vi "CycleVoltammetry.vi"() -> ()   [LabVIEW 2014]
uses:
  <vilib>/Instr/_visa.llb/VISA Configure Serial Port (Instr).vi
panel:
  in  "Combo Box":string(combo)
  out "R":dbl
  in  "stop":bool
  in  "file path (use dialog)":path
  in  "Title of experiment":string
  out "当前电流（A）":dbl
  out "Error buffer":string
  in  "Quiet Time Before SCAN(s)":dbl
  in  "VISA resource name":refnum<visa-resource-name>
  out "millisecond timer value 2":u32
  out "Index":dbl
  out "当前电压（V）":dbl
  in  "正向/反向(点亮)":bool
  out "V":dbl(graph)
  out "I":dbl(graph)
  out "I-U Graph":cluster{dbl[], dbl[]}(graph)
  in  "悬停（Pause）":bool
  out "Boolean":bool
  out "Run time":u32
  out "Program statement":string
  in  "Quiet Time(s)":dbl
  in  "反向/正向扫描(反向点亮)":bool caption="反向扫描"
  in  "Initial Voltage (起始电压\\V)":dbl
  in  "Sweep Segments(循环次数\\Times)":dbl
  out "Qutie Time （延时时间\\ms)":dbl
  in  "Low Voltage(最小电压\\V)":dbl
  in  "High Voltage(最大电压\\V)":dbl
  in  "Scan Rate(进步电压 V/Step）":dbl
  in  "Final Voltage(终止电压\\V)":dbl
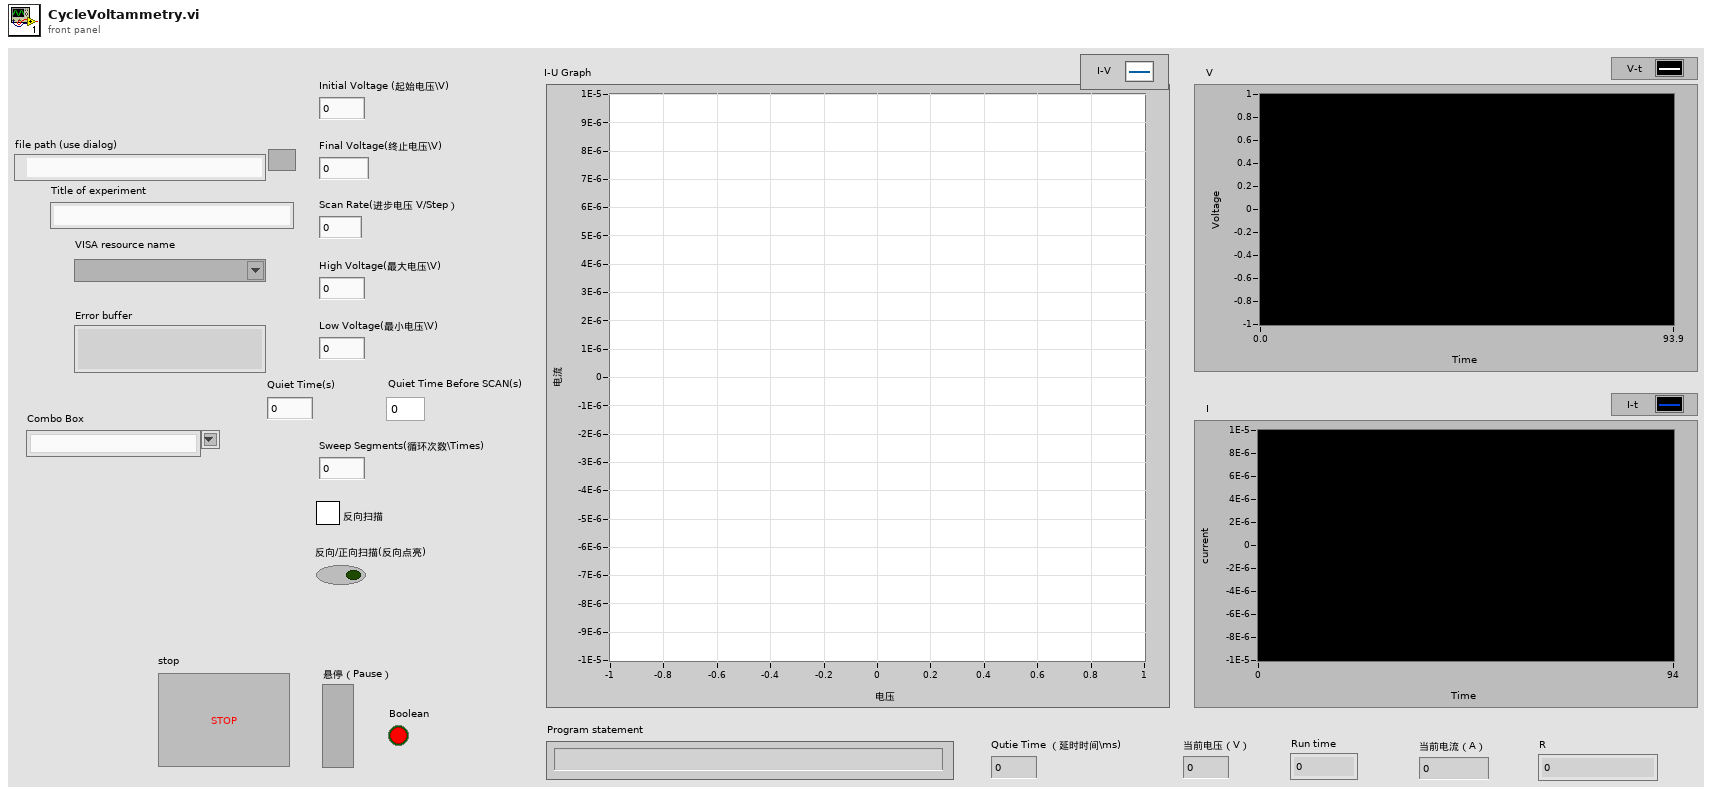
[diagram p1: front panel]
types:
  T1 = enum16{"open", "replace", "create", "open or create", "replace or create", "replace or create with confirmation"}
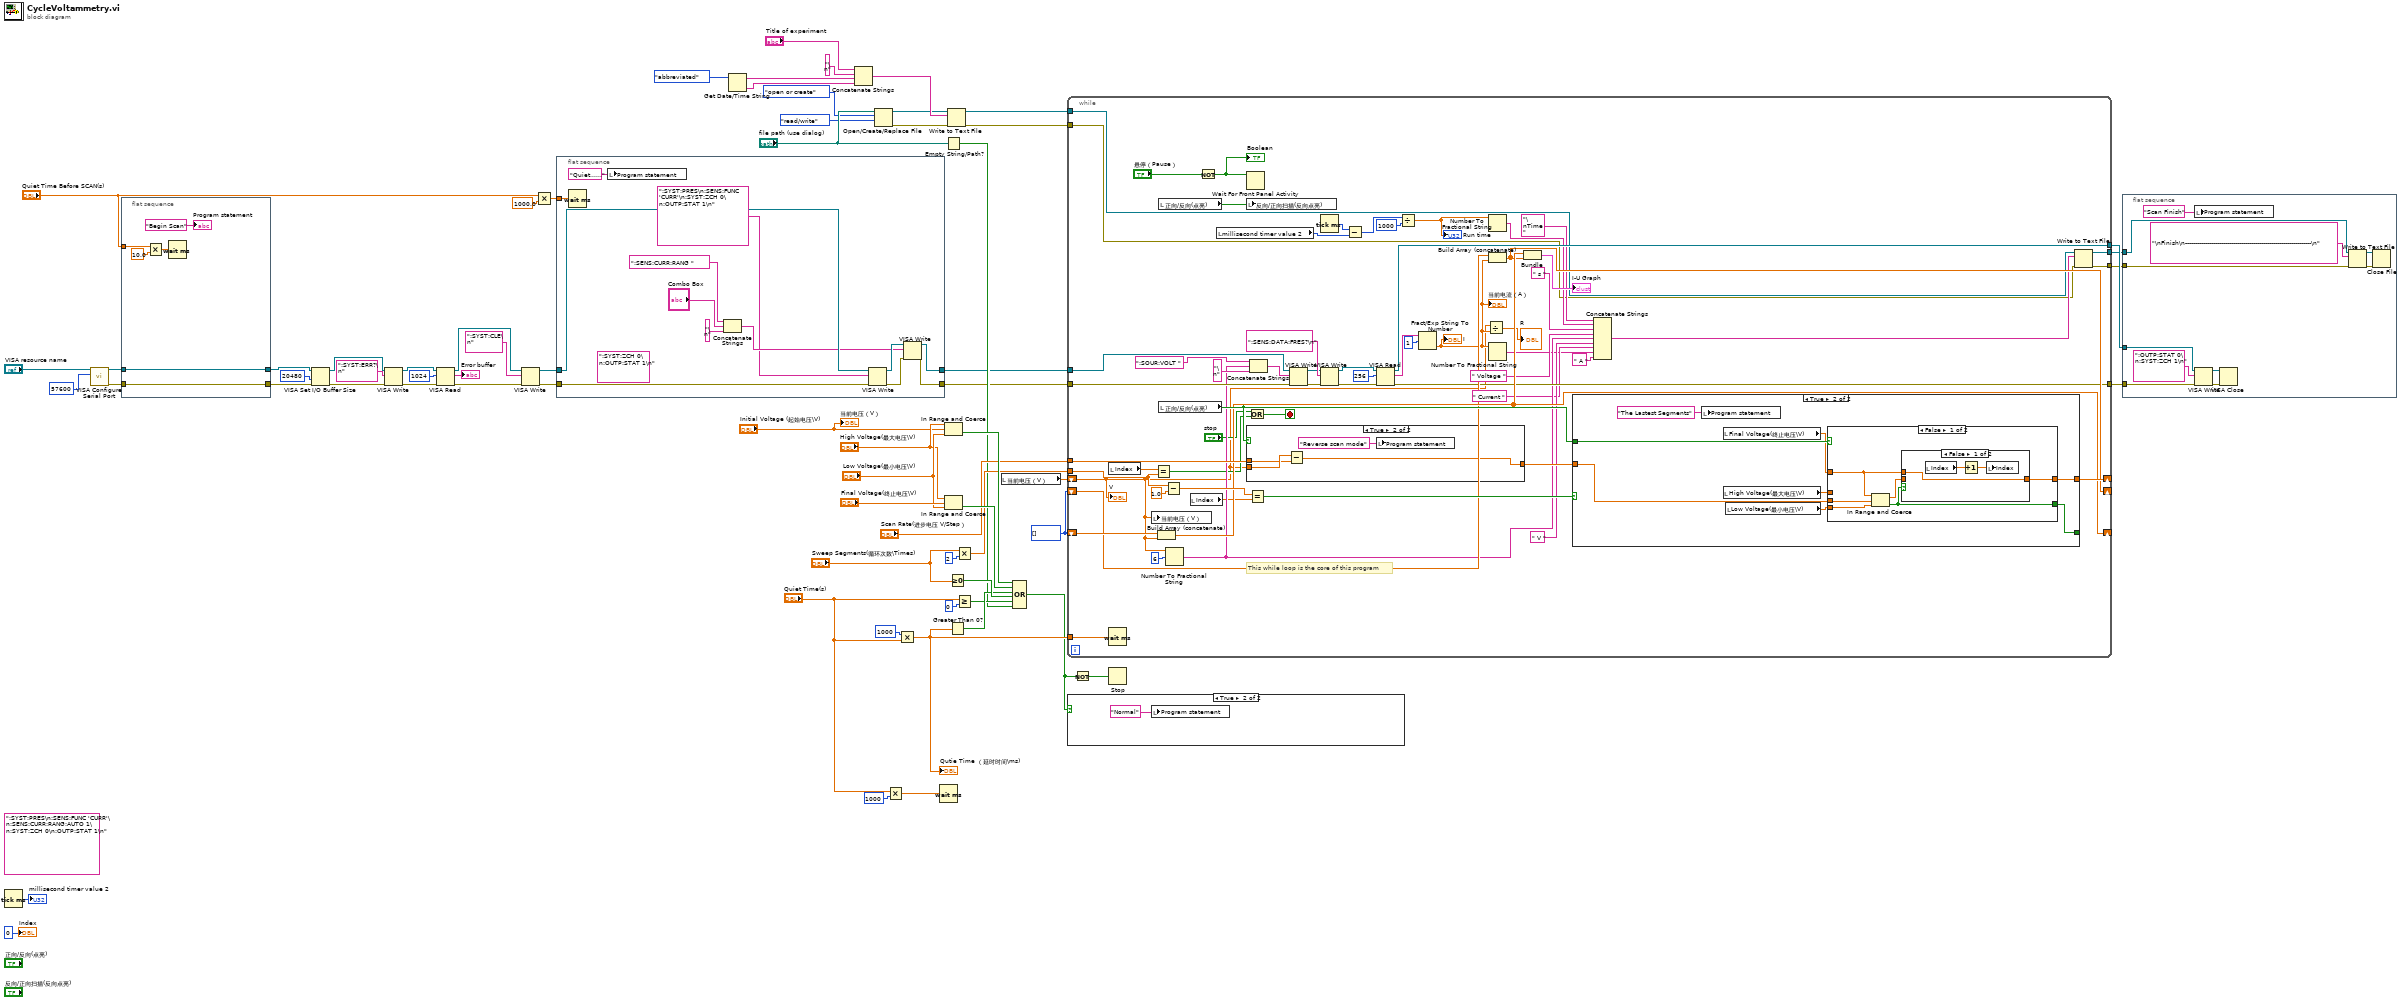
[diagram p0: block diagram]
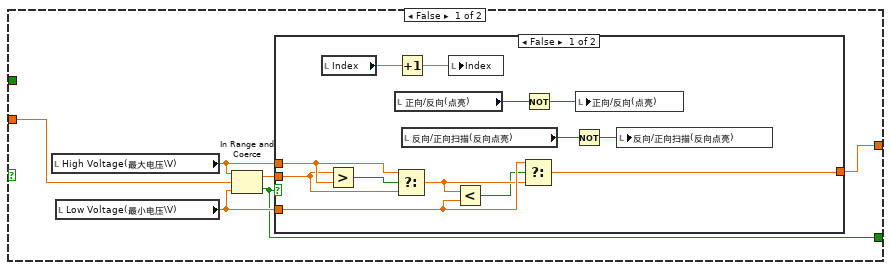
[diagram p2: hidden frame]
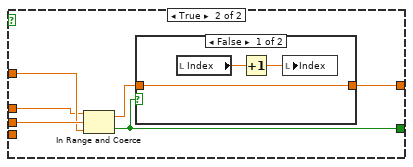
[diagram p5: hidden frame]
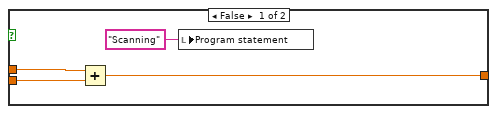
[diagram p7: hidden frame]
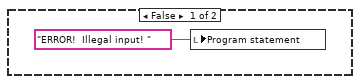
[diagram p8: hidden frame]
diagram:
  (unwired) ":SYST:PRES\n:SENS:FUNC 'CURR'\n:SENS:CURR:RANG:AUTO 1\n:SYST:ZCH 0\n:OUTP:STAT 1\n" ("write buffer")
  w46 = i32[] []
  n1 = Tick Count (ms)() -> (millisecond timer value=→"millisecond timer value 2":u32)
  n2 = call-poly "VISA Configure Serial Port"("VISA resource name"="VISA resource name", "baud rate (9600)"=u32 57600) -> ("VISA resource name out"=w13:refnum<visa-resource-name>, "error out"=w12:errorcluster)  [unwired: 12 in]
  n3 = flat-sequence {
    tunnel: [w72] -> w14
    tunnel: w13 -> [w72]
    tunnel: [w71] -> w11
    tunnel: w12 -> [w71]
    tunnel: "Quiet Time Before SCAN(s)" -> [w70]
    frame #0 {
      n4 = Multiply(x=w70, y=10.0) -> (x*y=w68:dbl)
      n5 = Wait (ms)(milliseconds to wait=w68) -> ()  [unwired: 1 out]
      "Program statement" <- "Begin Scan"
    }
  }
  n6 = VISA Set I/O Buffer Size(VISA resource name=w14, size (4096)=u32 20480, error in (no error)=w11) -> (VISA resource name out=w10:refnum<visa-resource-name>, error out=w9:errorcluster)  [unwired: 1 in]
  n7 = VISA Write(VISA resource name=w10, write buffer=":SYST:ERR?\n", error in (no error)=w9) -> (VISA resource name out=w40:refnum<visa-resource-name>, error out=w37:errorcluster)  [unwired: 1 out]
  n8 = VISA Read(VISA resource name=w40, byte count=u32 1024, error in (no error)=w37) -> (VISA resource name out=w35:refnum<visa-resource-name>, read buffer=→"Error buffer":string, error out=w34:errorcluster)  [unwired: 1 out]
  n9 = VISA Write(VISA resource name=w35, write buffer=":SYST:CLE\n", error in (no error)=w34) -> (VISA resource name out=w8:refnum<visa-resource-name>, error out=w5:errorcluster)  [unwired: 1 out]
  n10 = Multiply(x="Quiet Time Before SCAN(s)", y=1000.0) -> (x*y=w38:dbl)
  n11 = flat-sequence {
    tunnel: w38 -> [w86]
    tunnel: w8 -> [w84]
    tunnel: [w79] -> w7
    tunnel: [w78] -> w6
    tunnel: w5 -> [w83]
    frame #0 {
      (unwired) ":SYST:ZCH 0\n:OUTP:STAT 1\n" ("string")
      n12 = Wait (ms)(milliseconds to wait=w86) -> ()  [unwired: 1 out]
      n13 = local write "Program statement"("Quiet......") -> ()
      n14 = Concatenate Strings(":SENS:CURR:RANG " ("write buffer"), "Combo Box", "\n" ("string")) -> (w76:string)
      n15 = VISA Write(VISA resource name=w84, write buffer=":SYST:PRES\n:SENS:FUNC 'CURR'\n:SYST:ZCH 0\n:OUTP:STAT 1\n", error in (no error)=w83) -> (VISA resource name out=w80:refnum<visa-resource-name>, error out=w77:errorcluster)  [unwired: 1 out]
      n16 = VISA Write(VISA resource name=w80, write buffer=w76, error in (no error)=w77) -> (VISA resource name out=w79:refnum<visa-resource-name>, error out=w78:errorcluster)  [unwired: 1 out]
    }
  }
  n17 = Get Date/Time String(date format (0)=enum16{"short", "long", "abbreviated"}."abbreviated") -> (date string=w31:string, time string=w30:string)  [unwired: 2 in]
  n18 = Concatenate Strings("Title of experiment", "\n" ("string"), w31, w30) -> (w27:string)
  n19 = Open/Create/Replace File(file path (use dialog)="file path (use dialog)", operation (0:open)=T1."open or create", access (0:read/write)=enum16{"read/write", "read-only", "write-only"}."read/write") -> (refnum out=w26:refnum<file>, error out=w25:errorcluster)  [unwired: 3 in, 1 out]
  n20 = Multiply(x="Quiet Time(s)", y=1000) -> (x*y=w54:dbl)
  n21 = Multiply(x=1000, y="Quiet Time(s)") -> (x*y=w48:dbl)
  "Qutie Time （延时时间\\ms)" <- w48
  n22 = Wait (ms)(milliseconds to wait=w54) -> ()  [unwired: 1 out]
  n23 = In Range and Coerce(upper limit="High Voltage(最大电压\\V)", x="Initial Voltage (起始电压\\V)", lower limit="Low Voltage(最小电压\\V)") -> (In Range?=w64:bool)  [unwired: 1 out]
  n24 = In Range and Coerce(upper limit="High Voltage(最大电压\\V)", x="Final Voltage(终止电压\\V)", lower limit="Low Voltage(最小电压\\V)") -> (In Range?=w65:bool)  [unwired: 1 out]
  n25 = Empty String/Path?(string/path="file path (use dialog)") -> (empty?=w17:bool)
  n26 = Write to Text File(file (use dialog)=w26, text=w27, error in=w25) -> (refnum out=w24:refnum<file>, error out=w23:errorcluster)  [unwired: 1 in, 1 out]
  n27 = Greater Or Equal To 0?(x="Sweep Segments(循环次数\\Times)") -> (x >= 0?=w67:bool)
  n28 = Greater Than 0?(x=w48) -> (x > 0?=w66:bool)
  n29 = Multiply(x="Sweep Segments(循环次数\\Times)", y=2) -> (x*y=w50:dbl)
  n30 = Greater Or Equal?(x="Quiet Time(s)", y=0) -> (x >= y?=w57:bool)
  n31 = local read "当前电压（V）"() -> (w47:dbl)
  n32 = Compound Arithmetic op=OR(w64, w65, w66, w67, w57, w17) -> (w3:bool)
  n33 = while {
    tunnel: "Scan Rate(进步电压 V/Step）" -> [w146]
    shift-right: [w142] -> _
    shift-left: w47 -> [w87]
    tunnel: w48 -> [w145]
    tunnel: w50 -> [w92]
    shift-right: [w137] -> _
    shift-left: w46 -> [w138]
    shift-right: [w135] -> _
    shift-left: w46 -> [w136]
    tunnel: w7 -> [w123]
    tunnel: w6 -> [w122]
    tunnel: [w113] -> w21
    tunnel: [w112] -> w20
    tunnel: w24 -> [w100]
    tunnel: w23 -> [w99]
    tunnel: [w98] -> w16
    tunnel: [w97] -> w15
    stop <- w95 stop-if-true
    # "This while loop is the core of this program"
    n34 = local read "Index"() -> (w93:dbl)
    n35 = Wait (ms)(milliseconds to wait=w145) -> ()  [unwired: 1 out]
    n36 = local write "当前电压（V）"(w87) -> ()
    n37 = Equal?(x=w93, y=w92) -> (x = y?=w91:bool)
    n38 = Build Array (concatenate)(w138, w87) -> (w137:dbl[])
    n39 = local read "正向/反向(点亮)"() -> (w131:bool)
    n40 = local read "正向/反向(点亮)"() -> (w141:bool)
    n41 = Subtract(x=w92, y=1.0) -> (x-y=w140:dbl)
    n42 = Number To Fractional String(number=w87, width (-)=i16 6) -> (F-format string=w106:string)  [unwired: 2 in]
    n43 = local read "Index"() -> (w96:dbl)
    n44 = Not(x="悬停（Pause）") -> (.not. x?=w132:bool)
    "Boolean" <- w132
    n45 = local read "millisecond timer value 2"() -> (w129:u32)
    n46 = Wait For Front Panel Activity(3:w132) -> ()  [unwired: 2 in, 1 out]
    n47 = local write "反向/正向扫描(反向点亮)"(w131) -> ()
    n48 = case shown="True" w141 {
      tunnel: w146 -> [w198 w200]
      tunnel: w87 -> [w197 w201]
      tunnel: [w196 w199] -> w143
      frame False {
        n49 = Add(x=w198, y=w197) -> (x+y=w196:dbl)
        n50 = local write "Program statement"("Scanning") -> ()
      }
      frame True {
        n51 = Subtract(x=w201, y=w200) -> (x-y=w199:dbl)
        n52 = local write "Program statement"("Reverse scan mode") -> ()
      }
    }
    n53 = Or(x="stop", y=w91) -> (x .or. y?=w95:bool)
    n54 = Equal?(x=w140, y=w96) -> (x = y?=w144:bool)
    n55 = Concatenate Strings(":SOUR:VOLT " ("string"), w106, "\n" ("string")) -> (w124:string)
    n56 = VISA Write(VISA resource name=w123, write buffer=w124, error in (no error)=w122) -> (VISA resource name out=w120:refnum<visa-resource-name>, error out=w119:errorcluster)  [unwired: 1 out]
    n57 = Tick Count (ms)() -> (millisecond timer value=w130:u32)
    n58 = VISA Write(VISA resource name=w120, write buffer=":SENS:DATA:FRES?\n", error in (no error)=w119) -> (VISA resource name out=w117:refnum<visa-resource-name>, error out=w116:errorcluster)  [unwired: 1 out]
    n59 = Subtract(x=w130, y=w129) -> (x-y=w128:u32)
    n60 = VISA Read(VISA resource name=w117, byte count=u32 256, error in (no error)=w116) -> (VISA resource name out=w113:refnum<visa-resource-name>, read buffer=w115:string, error out=w112:errorcluster)  [unwired: 1 out]
    n61 = Divide(x=w128, y=u32 1000) -> (x/y=w110:dbl)
    "Run time" <- w110
    n62 = Fract/Exp String To Number(string=w115, offset=1) -> (number=w88:dbl)  [unwired: 2 in, 1 out]
    "I" <- w88
    "当前电流（A）" <- w88
    n63 = Divide(x=w87, y=w88) -> (x/y=→"R":dbl)
    n64 = Number To Fractional String(number=w110) -> (F-format string=w109:string)  [unwired: 3 in]
    n65 = Build Array (concatenate)(w136, w88) -> (w135:dbl[])
    n66 = Number To Fractional String(number=w88) -> (F-format string=w103:string)  [unwired: 3 in]
    n67 = Bundle(w137, w135) -> (→"I-U Graph":cluster{dbl[], dbl[]})  [unwired: 1 in]
    n68 = case shown="True" w144 {
      tunnel: w143 -> [w152 w168]
      tunnel: [w150 w171] -> w142
      tunnel: w141 -> [_ w174]
      tunnel: [w147 w170] -> _
      frame False {
        n69 = local read "High Voltage(最大电压\\V)"() -> (w149:dbl)
        n70 = local read "Low Voltage(最小电压\\V)"() -> (w148:dbl)
        n71 = In Range and Coerce(upper limit=w149, x=w152, lower limit=w148) -> (coerced(x)=w151:dbl, In Range?=w147:bool)
        n72 = case shown="False" w147 {
          tunnel: w151 -> [w158 w166]
          tunnel: [w161 w166] -> w150
          tunnel: w149 -> [w159 _]
          tunnel: w148 -> [w164 _]
          frame False {
            n73 = local read "Index"() -> (w157:dbl)
            n74 = Greater?(x=w158, y=w159) -> (0:w165:bool)
            n75 = local read "正向/反向(点亮)"() -> (w154:bool)
            n76 = Select(t=w159, s=w165, f=w158) -> (s? t:f=w163:dbl)
            n77 = Increment(x=w157) -> (x+1=w156:dbl)
            n78 = local read "反向/正向扫描(反向点亮)"() -> (w155:bool)
            n79 = local write "Index"(w156) -> ()
            n80 = Less?(x=w163, y=w164) -> (x < y?=w162:bool)
            n81 = Select(t=w164, s=w162, f=w163) -> (s? t:f=w161:dbl)
            n82 = Not(x=w154) -> (.not. x?=w153:bool)
            n83 = Not(x=w155) -> (.not. x?=w160:bool)
            n84 = local write "正向/反向(点亮)"(w153) -> ()
            n85 = local write "反向/正向扫描(反向点亮)"(w160) -> ()
          }
          frame True {
          }
        }
      }
      frame True {
        n86 = local write "Program statement"("The Lastest Segments") -> ()
        n87 = local read "Final Voltage(终止电压\\V)"() -> (w173:dbl)
        n88 = local read "High Voltage(最大电压\\V)"() -> (w169:dbl)
        n89 = local read "Low Voltage(最小电压\\V)"() -> (w172:dbl)
        n90 = case shown="False" w174 {
          tunnel: w173 -> [w175 w189]
          tunnel: w168 -> [w180 w190]
          tunnel: w172 -> [w179 _]
          tunnel: [w177 w187] -> w171
          tunnel: [w176 w186] -> w170
          tunnel: w169 -> [_ w188]
          frame False {
            n91 = In Range and Coerce(upper limit=w175, x=w180, lower limit=w179) -> (coerced(x)=w178:dbl, In Range?=w176:bool)
            n92 = case shown="False" w176 {
              tunnel: w178 -> [_ w184]
              tunnel: [w183 w184] -> w177
              tunnel: w175 -> [w183 _]
              frame False {
                n93 = local read "Index"() -> (w181:dbl)
                n94 = Increment(x=w181) -> (x+1=w182:dbl)
                n95 = local write "Index"(w182) -> ()
              }
              frame True {
              }
            }
          }
          frame True {
            n96 = In Range and Coerce(upper limit=w188, x=w190, lower limit=w189) -> (coerced(x)=w185:dbl, In Range?=w186:bool)
            n97 = case shown="False" w186 {
              tunnel: w185 -> [w193 w194]
              tunnel: [w193 w194] -> w187
              frame False {
                n98 = local read "Index"() -> (w191:dbl)
                n99 = Increment(x=w191) -> (x+1=w192:dbl)
                n100 = local write "Index"(w192) -> ()
              }
              frame True {
              }
            }
          }
        }
      }
    }
    n101 = Concatenate Strings("\nTime " ("string"), w109, " s " ("string"), " Voltage " ("string"), w106, " V " ("string"), " Current " ("string"), w103, " A " ("string")) -> (w101:string)
    n102 = Write to Text File(file (use dialog)=w100, text=w101, error in=w99) -> (refnum out=w98:refnum<file>, error out=w97:errorcluster)  [unwired: 1 in, 1 out]
    "V" <- w87
  }
  n103 = case shown="True" w3 {
    frame False {
      n104 = local write "Program statement"("ERROR!  Illegal input! ") -> ()
    }
    frame True {
      n105 = local write "Program statement"("Normal") -> ()
    }
  }
  n106 = Not(x=w3) -> (.not. x?=w59:bool)
  n107 = Stop(stop? (T)=w59) -> ()
  n108 = flat-sequence {
    tunnel: w21 -> [w212]
    tunnel: w20 -> [w211]
    tunnel: w16 -> [w206]
    tunnel: w15 -> [w205]
    frame #0 {
      n109 = local write "Program statement"("Scan Finish") -> ()
      n110 = VISA Write(VISA resource name=w212, write buffer=":OUTP:STAT 0\n:SYST:ZCH 1\n", error in (no error)=w211) -> (VISA resource name out=w213:refnum<visa-resource-name>, error out=w214:errorcluster)  [unwired: 1 out]
      n111 = VISA Close(VISA resource name=w213, error in (no error)=w214) -> ()  [unwired: 1 out]
      n112 = Write to Text File(file (use dialog)=w206, text="\nFinish\n---------------------------------------------------------------\n", error in=w205) -> (refnum out=w208:refnum<file>, error out=w207:errorcluster)  [unwired: 1 in, 1 out]
      n113 = Close File(refnum=w208, error in=w207) -> ()  [unwired: 2 out]
    }
  }
  "当前电压（V）" <- "Initial Voltage (起始电压\\V)"
  "Index" <- 0
